vi "Version_2.0_Single_Column_Code.vi"() -> ()   [LabVIEW 2020] (continued)
                                n1436 = local read "VISA Refnum in\nfor Pump"() -> (w1853:refnum<visa-resource-name>)
                                n1437 = case shown="True" w1852 {
                                frame False {
                                }
                                frame True {
                                n1438 = local read "VISA Refnum in\nfor Pump"() -> (w1854:refnum<visa-resource-name>)
                                n1439 = call "HardStopCurrentProcess (SubVI).vi"("VISA Refnum in"=w1854) -> ()  [unwired: 11 in]
                                }
                                }
                                n1440 = call "ProcessCompletionWaiter (SubVI).vi"("VISA Refnum in"=w1853) -> ()  [unwired: 11 in]
                                }
                                }
                                }
                              }
                            }
                          }
                          frame #3 {
                            n1441 = local read "VISA Refnum in\nfor Pump"() -> (w1856:refnum<visa-resource-name>)
                            n1442 = local read "Port for \nB-Elution"() -> (w1855:string)
                            n1443 = call "PortChanger (SubVI).vi"("Port Number"=w1855, "VISA Refnum in"=w1856) -> ()  [unwired: 10 in]
                          }
                          frame #4 {
                            n1444 = local read "VISA Refnum in\nfor Pump"() -> (w1857:refnum<visa-resource-name>)
                            n1445 = call "ProcessCompletionWaiter (SubVI).vi"("VISA Refnum in"=w1857) -> ()  [unwired: 11 in]
                          }
                          frame #5 {
                            n1446 = local read "Buffer-B PickUp \nFlow Rate (ul/min)"() -> (w1860:dbl)
                            n1447 = local read "Buffer-B Pumping\nResolution"() -> (w1859:T2)
                            n1448 = local read "VISA Refnum in\nfor Pump"() -> (w1862:refnum<visa-resource-name>)
                            n1449 = local read "Buffer-B Volume \nto be  Pumped"() -> (w1858:dbl)
                            n1450 = local read "Volume of Syringe"() -> (w1861:dbl)
                            n1451 = call "RPickUp(SubVI).vi"("Volume to be picked up"=w1858, "Volume of Syringe"=w1861, "Resolution of PickUP"=w1859, "PickUp Flow Rate (ul/min)"=w1860, "VISA Refnum in"=w1862) -> ()  [unwired: 6 in, 1 out]
                          }
                          frame #6 {
                            n1452 = local read "Stopper that ends \nthe main loops"() -> (w1863:bool)
                            n1453 = local read "VISA Refnum in\nfor Pump"() -> (w1864:refnum<visa-resource-name>)
                            n1454 = case shown="True" w1863 {
                              frame False {
                              }
                              frame True {
                                n1455 = local read "VISA Refnum in\nfor Pump"() -> (w1865:refnum<visa-resource-name>)
                                n1456 = call "HardStopCurrentProcess (SubVI).vi"("VISA Refnum in"=w1865) -> ()  [unwired: 11 in]
                              }
                            }
                            n1457 = call "ProcessCompletionWaiter (SubVI).vi"("VISA Refnum in"=w1864) -> ()  [unwired: 11 in]
                          }
                          frame #7 {
                            # "Reads the initial Plunger Position for computing the volume dispensed"
                            n1458 = local read "VISA Refnum in\nfor Pump"() -> (w1867:refnum<visa-resource-name>)
                            n1459 = call "AbsolutePlungerPosition (SubVI).vi"("VISA Refnum in"=w1867) -> ("Plunger Position"=w1866:i32)  [unwired: 10 in]
                            n1460 = local write "Initial Plunger Position"(w1866) -> ()
                          }
                          frame #8 {
                            # "Switch to Port-2"
                            # "Port-2 of the pump is conncted to column-1 of chip"
                            n1461 = local read "VISA Refnum in\nfor Pump"() -> (w1869:refnum<visa-resource-name>)
                            n1462 = call "PortChanger (SubVI).vi"("Port Number"="2", "VISA Refnum in"=w1869) -> ()  [unwired: 10 in]
                          }
                          frame #9 {
                            n1463 = local read "Stopper that ends \nthe main loops"() -> (w1870:bool)
                            n1464 = local read "VISA Refnum in\nfor Pump"() -> (w1871:refnum<visa-resource-name>)
                            n1465 = case shown="True" w1870 {
                              frame False {
                              }
                              frame True {
                                n1466 = local read "VISA Refnum in\nfor Pump"() -> (w1872:refnum<visa-resource-name>)
                                n1467 = call "HardStopCurrentProcess (SubVI).vi"("VISA Refnum in"=w1872) -> ()  [unwired: 11 in]
                              }
                            }
                            n1468 = call "ProcessCompletionWaiter (SubVI).vi"("VISA Refnum in"=w1871) -> ()  [unwired: 11 in]
                          }
                          frame #10 {
                            # "Keeps the AMF valve after column-1 open and valve after column-2 closed"
                            n1469 = local read "VISA Refnum in\nfor Valve"() -> (w1877:refnum<visa-resource-name>)
                            n1470 = local read "External Valve \nOPEN"() -> (w1876:string)
                            n1471 = call "PortChanger_Valve (SubVI).vi"("Port Number"=w1876, "VISA Refnum in"=w1877) -> ()  [unwired: 10 in]
                            n1472 = local write "Valve V1 Open"(TRUE ("Valve V1 Open")) -> ()
                            n1473 = local write "Valve V2 Open"(TRUE ("Valve V2 Open")) -> ()
                            n1474 = local write "Valve V3 Open"(FALSE ("Valve V3 Open")) -> ()
                            n1475 = local write "Valve V4 Open"(FALSE ("Valve V4 Open")) -> ()
                            n1476 = local write "Valve V6 Open"(FALSE ("Valve V6 Open")) -> ()
                            n1477 = local write "Valve V5 Open"(FALSE ("Valve V5 Open")) -> ()
                            n1478 = local write "Valve V7 Open"(FALSE ("Valve V7 Open")) -> ()
                          }
                          frame #11 {
                            n1479 = local read "Buffer-B Dispense\nFlow Rate (ul/min)"() -> (w1887:dbl)
                            n1480 = local read "Buffer-B Pumping\nResolution"() -> (w1886:T2)
                            n1481 = local read "Initial Plunger Position"() -> (w1883:dbl)
                            n1482 = local read "VISA Refnum in\nfor Pump"() -> (w1889:refnum<visa-resource-name>)
                            n1483 = local read "Volume of Syringe"() -> (w1888:dbl)
                            n1484 = call "GoToAbsolutePosition(SubVI).vi"("Absolute Volume Position in Syringe (in ul)"=0.0 ("Volume to be Dispensed"), "Volume of Syringe"=w1888, "Resolution of Pumping"=w1886, "Flow Rate (ul/min)"=w1887, "VISA Refnum in"=w1889) -> ()  [unwired: 6 in, 1 out]
                            n1485 = local write "Pause Data Collection"(FALSE ("Pause Data Collection")) -> ()
                            n1486 = local write "Vol_now"(0.0 ("Vol_now")) -> ()
                            n1487 = local write "Position\nNow"(w1883) -> ()
                          }
                          frame #12 {
                            n1488 = while {
                              stop <- w1896 stop-if-true
                              n1489 = event shown="[1] Timeout" {
                                selector: _ -> [_ _]
                                dyn-events: _ -> [_ _]
                                timeout: 100 -> [_ _]
                                event "Pause Elution\nValue": Value Change {
                                n1490 = event-data() -> ()  [unwired: 1 in, 6 out]
                                n1491 = stacked-sequence {
                                frame #0 {
                                n1492 = local read "Pause Elution"() -> (w1898:bool)
                                n1493 = case shown="False" w1898 {
                                frame False {
                                n1494 = local write "Pause Elution"(TRUE ("Pause Elution")) -> ()
                                }
                                frame True {
                                n1495 = local write "Pause Elution"(FALSE ("Pause Elution")) -> ()
                                }
                                }
                                }
                                frame #1 {
                                n1496 = local read "Pause Elution"() -> (w1901:bool)
                                n1497 = case shown="False" w1901 {
                                frame False {
                                n1498 = local read "Buffer-B Dispense\nFlow Rate (ul/min)"() -> (w1906:dbl)
                                n1499 = local read "VISA Refnum in\nfor Pump"() -> (w1907:refnum<visa-resource-name>)
                                n1500 = local read "Buffer-B Pumping\nResolution"() -> (w1903:T2)
                                n1501 = local read "Volume of Syringe"() -> (w1904:dbl)
                                n1502 = call "GoToAbsolutePosition(SubVI).vi"("Absolute Volume Position in Syringe (in ul)"=0.0, "Volume of Syringe"=w1904, "Resolution of Pumping"=w1903, "Flow Rate (ul/min)"=w1906, "VISA Refnum in"=w1907) -> ()  [unwired: 6 in, 1 out]
                                n1503 = local write "Pause Data Collection"(FALSE ("Pause Data Collection")) -> ()
                                }
                                frame True {
                                n1504 = local read "VISA Refnum in\nfor Pump"() -> (w1909:refnum<visa-resource-name>)
                                n1505 = local write "Pause Data Collection"(TRUE ("Pause Data Collection")) -> ()
                                n1506 = call "HardStopCurrentProcess (SubVI).vi"("VISA Refnum in"=w1909) -> ()  [unwired: 11 in]
                                }
                                }
                                }
                                }
                                }
                                event Timeout {
                                n1507 = event-data() -> ()  [unwired: 1 in, 3 out]
                                }
                              }
                              n1508 = local read "Stopper that ends \nthe main loops"() -> (w1895:bool)
                              n1509 = local read "Divert Sample \ninto Column-2"() -> (w1894:bool)
                              n1510 = Or(x=w1894, y=w1895) -> (x .or. y?=w1896:bool)
                            }
                            n1511 = local read "Buffer-B Pumping\nResolution"() -> (w1892:T2)
                            n1512 = local read "VISA Refnum in\nfor Pump"() -> (w1893:refnum<visa-resource-name>)
                            n1513 = local read "Volume of Syringe"() -> (w1891:dbl)
                            n1514 = while {
                              tunnel: w1893 -> [w1918]
                              tunnel: w1892 -> [w1917]
                              tunnel: w1891 -> [w1916]
                              stop <- w1912 stop-if-true
                              n1515 = local read "Position\nNow"() -> (w1910:dbl)
                              n1516 = local read "Pause Elution"() -> (w1911:bool)
                              n1517 = case shown="True" w1911 {
                                tunnel: w1910 -> [w1922 _]
                                tunnel: w1918 -> [w1921 w1964]
                                tunnel: w1917 -> [w1920 _]
                                tunnel: w1916 -> [w1919 _]
                                frame False {
                                n1518 = stacked-sequence {
                                tunnel: w1922 -> [_ w1928]
                                tunnel: w1921 -> [_ w1927]
                                tunnel: w1920 -> [_ w1926]
                                tunnel: w1919 -> [_ w1925]
                                frame #0 {
                                n1519 = Wait (ms)(milliseconds to wait=u32 3000) -> ()  [unwired: 1 out]
                                n1520 = local write "Signal"(TRUE ("Signal")) -> ()
                                }
                                frame #1 {
                                n1521 = while {
                                tunnel: w1928 -> [w1940]
                                tunnel: w1927 -> [w1939]
                                tunnel: w1926 -> [w1938]
                                tunnel: w1925 -> [w1937]
                                stop <- w1932 stop-if-true
                                n1522 = stacked-sequence {
                                tunnel: w1940 -> [_ w1947]
                                tunnel: w1939 -> [_ w1946]
                                tunnel: w1938 -> [_ w1945]
                                tunnel: w1937 -> [_ w1944]
                                frame #0 {
                                n1523 = Wait (ms)(milliseconds to wait=u32 500) -> ()  [unwired: 1 out]
                                }
                                frame #1 {
                                n1524 = call "AbsolutePlungerPosition (SubVI).vi"("VISA Refnum in"=w1946) -> ("Plunger Position"=w1943:i32)  [unwired: 10 in]
                                n1525 = case shown="\"High Resolution Pumping\"" w1945 {
                                tunnel: w1947 -> [w1952 w1961]
                                tunnel: w1943 -> [w1953 w1960]
                                tunnel: [w1951 w1958] -> w1942
                                tunnel: w1944 -> [w1950 w1959]
                                frame "Standard Pumping", Default {
                                n1526 = Subtract(x=w1952, y=w1953) -> (x-y=w1949:dbl)
                                n1527 = Absolute Value(x=w1949) -> (abs(x)=w1948:dbl)
                                n1528 = Multiply(x=w1948, y=w1950) -> (x*y=w1955:dbl)
                                n1529 = Divide(x=w1955, y=3000.0) -> (x/y=w1951:dbl)
                                }
                                frame "High Resolution Pumping" {
                                n1530 = Subtract(x=w1961, y=w1960) -> (x-y=w1957:dbl)
                                n1531 = Absolute Value(x=w1957) -> (abs(x)=w1956:dbl)
                                n1532 = Multiply(x=w1956, y=w1959) -> (x*y=w1963:dbl)
                                n1533 = Divide(x=w1963, y=24000.0) -> (x/y=w1958:dbl)
                                }
                                }
                                n1534 = local write "Volume being Injected \nin this process"(w1942) -> ()
                                }
                                }
                                n1535 = local read "Volume being Injected \nin this process"() -> (w1930:dbl)
                                n1536 = local read "Affinity Elution \nGraph Min CutOff"() -> (w1929:dbl)
                                n1537 = local read "Stopper that ends \nthe main loops"() -> (w1935:bool)
                                n1538 = local read "Divert Sample \ninto Column-2"() -> (w1936:bool)
                                n1539 = Greater Or Equal?(x=w1930, y=w1929) -> (x >= y?=w1931:bool)
                                n1540 = Or(x=w1936, y=w1935) -> (x .or. y?=w1933:bool)
                                n1541 = local read "Pause Elution"() -> (w1934:bool)
                                n1542 = local write "Affinity Elution \nis Approaching"(w1931) -> ()
                                n1543 = Or(x=w1934, y=w1933) -> (x .or. y?=w1932:bool)
                                }
                                }
                                }
                                }
                                frame True {
                                n1544 = stacked-sequence {
                                tunnel: w1964 -> [_ w1967 _]
                                frame #0 {
                                n1545 = Wait (ms)(milliseconds to wait=u32 2000) -> ()  [unwired: 1 out]
                                }
                                frame #1 {
                                n1546 = local read "Signal"() -> (w1966:bool)
                                n1547 = case shown="True" w1966 {
                                tunnel: w1967 -> [_ w1973]
                                frame False {
                                }
                                frame True {
                                n1548 = local read "Volume being Injected \nin this process"() -> (w1971:dbl)
                                n1549 = local read "Net Elution \nVolume"() -> (w1970:dbl)
                                n1550 = local write "Signal"(FALSE ("Signal")) -> ()
                                n1551 = Add(x=w1971, y=w1970) -> (x+y=w1969:dbl)
                                n1552 = call "AbsolutePlungerPosition (SubVI).vi"("VISA Refnum in"=w1973) -> ("Plunger Position"=w1972:i32)  [unwired: 10 in]
                                n1553 = local write "Net Elution \nVolume"(w1969) -> ()
                                n1554 = local write "Position\nNow"(w1972) -> ()
                                }
                                }
                                }
                                frame #2 {
                                n1555 = local write "Volume being Injected \nin this process"(0.0 ("Volume being Injected \nin this process")) -> ()
                                }
                                }
                                }
                              }
                              n1556 = local read "Stopper that ends \nthe main loops"() -> (w1914:bool)
                              n1557 = local read "Divert Sample \ninto Column-2"() -> (w1913:bool)
                              n1558 = Or(x=w1913, y=w1914) -> (x .or. y?=w1912:bool)
                              n1559 = Wait (ms)(milliseconds to wait=u32 300) -> ()  [unwired: 1 out]
                            }
                            n1560 = local read "Stopper that ends \nthe main loops"() -> (w1890:bool)
                            n1561 = case shown="True" w1890 {
                              frame False {
                              }
                              frame True {
                                n1562 = local read "VISA Refnum in\nfor Pump"() -> (w1975:refnum<visa-resource-name>)
                                n1563 = call "HardStopCurrentProcess (SubVI).vi"("VISA Refnum in"=w1975) -> ()  [unwired: 11 in]
                              }
                            }
                          }
                          frame #13 {
                            # "valve after column-1 is closed"
                            # "Keeps the on-chip Valve V1 and V3 after column-2 open"
                            # "Keeps the AMF valve after column-1 closed and valve after column-2 open"
                            n1564 = local read "VISA Refnum in\nfor Pump"() -> (w1988:refnum<visa-resource-name>)
                            n1565 = local read "Volume being Injected \nin this process"() -> (w1985:dbl)
                            n1566 = local write "Sample Volume Diverted\ninto Column-2"(0.0 ("Sample Volume Diverted\ninto Column-2")) -> ()
                            n1567 = call "AbsolutePlungerPosition (SubVI).vi"("VISA Refnum in"=w1988) -> ("Plunger Position"=w1987:i32)  [unwired: 10 in]
                            n1568 = local write "Position\nNow"(w1987) -> ()
                            n1569 = local write "Vol_previous"(0.0 ("Vol_diff")) -> ()
                            n1570 = local write "Vol_now"(w1985) -> ()
                            n1571 = local read "VISA Refnum in\nfor Valve"() -> (w1980:refnum<visa-resource-name>)
                            n1572 = local read "External Valve \nCLOSED"() -> (w1979:string)
                            n1573 = local write "Valve V1 Open"(TRUE ("Valve V1 Open")) -> ()
                            n1574 = local write "Valve V3 Open"(TRUE ("Valve V3 Open")) -> ()
                            n1575 = local write "Valve V2 Open"(FALSE ("Valve V2 Open")) -> ()
                            n1576 = local write "Valve V4 Open"(TRUE ("Valve V4 Open")) -> ()
                            n1577 = call "PortChanger_Valve (SubVI).vi"("Port Number"=w1979, "VISA Refnum in"=w1980) -> ()  [unwired: 10 in]
                            n1578 = local write "Valve V5 Open"(TRUE ("Valve V5 Open")) -> ()
                            n1579 = local write "Valve V6 Open"(FALSE ("Valve V6 Open")) -> ()
                            n1580 = local write "Valve V7 Open"(TRUE ("Valve V7 Open")) -> ()
                          }
                          frame #14 {
                            n1581 = local read "Divert Sample \ninto Column-2"() -> (w1990:bool)
                            n1582 = case shown="True" w1990 {
                              frame False {
                                n1583 = stacked-sequence {
                                frame #0 {
                                n1584 = local read "Buffer-B Pumping\nResolution"() -> (w1993:T2)
                                n1585 = local read "VISA Refnum in\nfor Pump"() -> (w1995:refnum<visa-resource-name>)
                                n1586 = local read "Initial Plunger Position"() -> (w1994:dbl)
                                n1587 = local read "Volume of Syringe"() -> (w1992:dbl)
                                n1588 = while {
                                tunnel: w1994 -> [w2001]
                                tunnel: w1995 -> [w2000]
                                tunnel: w1993 -> [w1999]
                                tunnel: w1992 -> [w1998]
                                stop <- w1996 stop-if-true
                                n1589 = Wait (ms)(milliseconds to wait=u32 100) -> ()  [unwired: 1 out]
                                n1590 = stacked-sequence {
                                tunnel: w2001 -> [w2007 _]
                                tunnel: w2000 -> [w2006 w2027]
                                tunnel: w1999 -> [w2005 _]
                                tunnel: w1998 -> [w2004 _]
                                tunnel: [_ w2025] -> w1996
                                frame #0 {
                                n1591 = call "AbsolutePlungerPosition (SubVI).vi"("VISA Refnum in"=w2006) -> ("Plunger Position"=w2003:i32)  [unwired: 10 in]
                                n1592 = case shown="\"Standard Pumping\", Default" w2005 {
                                tunnel: w2007 -> [w2012 w2021]
                                tunnel: w2003 -> [w2013 w2020]
                                tunnel: [w2011 w2018] -> w2002
                                tunnel: w2004 -> [w2010 w2019]
                                frame "Standard Pumping", Default {
                                n1593 = Subtract(x=w2012, y=w2013) -> (x-y=w2009:dbl)
                                n1594 = Absolute Value(x=w2009) -> (abs(x)=w2008:dbl)
                                n1595 = Multiply(x=w2008, y=w2010) -> (x*y=w2015:dbl)
                                n1596 = Divide(x=w2015, y=3000.0) -> (x/y=w2011:dbl)
                                }
                                frame "High Resolution Pumping" {
                                n1597 = Subtract(x=w2021, y=w2020) -> (x-y=w2017:dbl)
                                n1598 = Absolute Value(x=w2017) -> (abs(x)=w2016:dbl)
                                n1599 = Multiply(x=w2016, y=w2019) -> (x*y=w2023:dbl)
                                n1600 = Divide(x=w2023, y=24000.0) -> (x/y=w2018:dbl)
                                }
                                }
                                n1601 = local write "Volume being Injected \nin this process"(w2002) -> ()
                                }
                                frame #1 {
                                n1602 = local read "Stopper that ends \nthe main loops"() -> (w2024:bool)
                                n1603 = call "LSPOneStatus (SubVI).vi"("VISA Refnum in"=w2027) -> ("read buffer"=w2029:string)  [unwired: 10 in]
                                n1604 = call <vilib>:"Trim Whitespace.vi"("string"=w2029) -> ("trimmed string"=w2028:string)  [unwired: 1 in]
                                n1605 = Equal?(x=w2028, y="/0`\u0003") -> (x = y?=w2026:bool)
                                n1606 = Or(x=w2026, y=w2024) -> (x .or. y?=w2025:bool)
                                }
                                }
                                }
                                n1607 = local read "Stopper that ends \nthe main loops"() -> (w1991:bool)
                                n1608 = case shown="True" w1991 {
                                frame False {
                                }
                                frame True {
                                n1609 = local read "VISA Refnum in\nfor Pump"() -> (w2031:refnum<visa-resource-name>)
                                n1610 = call "HardStopCurrentProcess (SubVI).vi"("VISA Refnum in"=w2031) -> ()  [unwired: 11 in]
                                }
                                }
                                }
                                }
                              }
                              frame True {
                                n1611 = stacked-sequence {
                                frame #0 {
                                n1612 = local read "Buffer-B Pumping\nResolution"() -> (w2034:T2)
                                n1613 = local read "VISA Refnum in\nfor Pump"() -> (w2036:refnum<visa-resource-name>)
                                n1614 = local read "Volume of Syringe"() -> (w2033:dbl)
                                n1615 = local read "Position\nNow"() -> (w2035:dbl)
                                n1616 = while {
                                tunnel: w2035 -> [w2042]
                                tunnel: w2036 -> [w2041]
                                tunnel: w2034 -> [w2040]
                                tunnel: w2033 -> [w2039]
                                stop <- w2037 stop-if-true
                                n1617 = Wait (ms)(milliseconds to wait=u32 100) -> ()  [unwired: 1 out]
                                n1618 = stacked-sequence {
                                tunnel: w2042 -> [w2052 _ _]
                                tunnel: w2041 -> [w2051 _ w2078]
                                tunnel: w2040 -> [w2050 _ _]
                                tunnel: w2039 -> [w2049 _ _]
                                tunnel: [_ _ w2076] -> w2037
                                frame #0 {
                                n1619 = local read "Vol_previous"() -> (w2046:dbl)
                                n1620 = call "AbsolutePlungerPosition (SubVI).vi"("VISA Refnum in"=w2051) -> ("Plunger Position"=w2048:i32)  [unwired: 10 in]
                                n1621 = case shown="\"Standard Pumping\", Default" w2050 {
                                tunnel: w2052 -> [w2057 w2066]
                                tunnel: w2048 -> [w2058 w2065]
                                tunnel: [w2056 w2063] -> w2047
                                tunnel: w2049 -> [w2055 w2064]
                                frame "Standard Pumping", Default {
                                n1622 = Subtract(x=w2057, y=w2058) -> (x-y=w2054:dbl)
                                n1623 = Absolute Value(x=w2054) -> (abs(x)=w2053:dbl)
                                n1624 = Multiply(x=w2053, y=w2055) -> (x*y=w2060:dbl)
                                n1625 = Divide(x=w2060, y=3000.0) -> (x/y=w2056:dbl)
                                }
                                frame "High Resolution Pumping" {
                                n1626 = Subtract(x=w2066, y=w2065) -> (x-y=w2062:dbl)
                                n1627 = Absolute Value(x=w2062) -> (abs(x)=w2061:dbl)
                                n1628 = Multiply(x=w2061, y=w2064) -> (x*y=w2068:dbl)
                                n1629 = Divide(x=w2068, y=24000.0) -> (x/y=w2063:dbl)
                                }
                                }
                                n1630 = Subtract(x=w2047, y=w2046) -> (x-y=w2045:dbl)
                                n1631 = local read "Vol_now"() -> (w2043:dbl)
                                n1632 = local write "Sample Volume Diverted\ninto Column-2"(w2047) -> ()
                                n1633 = Add(x=w2045, y=w2043) -> (x+y=w2044:dbl)
                                n1634 = local write "Volume being Injected \nin this process"(w2044) -> ()
                                }
                                frame #1 {
                                n1635 = local read "Volume being Injected \nin this process"() -> (w2069:dbl)
                                n1636 = local read "Sample Volume Diverted\ninto Column-2"() -> (w2070:dbl)
                                n1637 = local write "Vol_now"(w2069) -> ()
                                n1638 = local write "Vol_previous"(w2070) -> ()
                                }
                                frame #2 {
                                n1639 = local read "Buffer-B Volume \nto be Pumped for\nSample Diversion\nto Column-2"() -> (w2072:dbl)
                                n1640 = local read "Sample Volume Diverted\ninto Column-2"() -> (w2071:dbl)
                                n1641 = local read "Stopper that ends \nthe main loops"() -> (w2073:bool)
                                n1642 = call "LSPOneStatus (SubVI).vi"("VISA Refnum in"=w2078) -> ("read buffer"=w2080:string)  [unwired: 10 in]
                                n1643 = call <vilib>:"Trim Whitespace.vi"("string"=w2080) -> ("trimmed string"=w2079:string)  [unwired: 1 in]
                                n1644 = Equal?(x=w2079, y="/0`\u0003") -> (x = y?=w2077:bool)
                                n1645 = Greater Or Equal?(x=w2071, y=w2072) -> (x >= y?=w2075:bool)
                                n1646 = Or(x=w2073, y=w2075) -> (x .or. y?=w2074:bool)
                                n1647 = Or(x=w2077, y=w2074) -> (x .or. y?=w2076:bool)
                                }
                                }
                                }
                                n1648 = local read "Stopper that ends \nthe main loops"() -> (w2032:bool)
                                n1649 = case shown="True" w2032 {
                                frame False {
                                }
                                frame True {
                                n1650 = local read "VISA Refnum in\nfor Pump"() -> (w2082:refnum<visa-resource-name>)
                                n1651 = call "HardStopCurrentProcess (SubVI).vi"("VISA Refnum in"=w2082) -> ()  [unwired: 11 in]
                                }
                                }
                                }
                                frame #1 {
                                n1652 = local read "VISA Refnum in\nfor Pump"() -> (w2084:refnum<visa-resource-name>)
                                n1653 = local write "Pause Data Collection"(TRUE ("Pause Data Collection")) -> ()
                                n1654 = call "HardStopCurrentProcess (SubVI).vi"("VISA Refnum in"=w2084) -> ()  [unwired: 11 in]
                                }
                                frame #2 {
                                n1655 = local read "VISA Refnum in\nfor Pump"() -> (w2085:refnum<visa-resource-name>)
                                n1656 = call "PortChanger (SubVI).vi"("Port Number"="1", "VISA Refnum in"=w2085) -> ()  [unwired: 10 in]
                                }
                                frame #3 {
                                n1657 = local read "VISA Refnum in\nfor Pump"() -> (w2091:refnum<visa-resource-name>)
                                n1658 = local read "Volume of Syringe"() -> (w2087:dbl)
                                n1659 = call "GoToAbsolutePosition(SubVI).vi"("Absolute Volume Position in Syringe (in ul)"=0.0, "Volume of Syringe"=w2087, "Resolution of Pumping"=T2."Standard Pumping", "Flow Rate (ul/min)"=150.0, "VISA Refnum in"=w2091) -> ()  [unwired: 6 in, 1 out]
                                }
                                frame #4 {
                                n1660 = local read "VISA Refnum in\nfor Pump"() -> (w2093:refnum<visa-resource-name>)
                                n1661 = local write "Divert Sample \ninto Column-2"(FALSE ("Divert Sample \ninto Column-2")) -> ()
                                n1662 = call "ProcessCompletionWaiter (SubVI).vi"("VISA Refnum in"=w2093) -> ()  [unwired: 11 in]
                                }
                                }
                              }
                            }
                          }
                          frame #15 {
                            # "Keeps the On-Chip Valves V1 and V3 closed"
                            # "Switch to Port-5/8"
                            # "Port-5/8 of pump is connected to Buffer-C1/C2"
                            # "Keeps the AMF valve after column-1 open and valve after column-2 closed"
                            n1663 = local read "VISA Refnum in\nfor Pump"() -> (w2106:refnum<visa-resource-name>)
                            n1664 = local write "Pause Data Collection"(TRUE ("Pause Data Collection")) -> ()
                            n1665 = Wait (ms)(milliseconds to wait=u32 500) -> ()  [unwired: 1 out]
                            n1666 = local write "Affinity On"(FALSE ("Affinity On")) -> ()
                            n1667 = local read "Port for \nC2-Elution"() -> (w2097:string)
                            n1668 = local write "Affinity Elution On"(FALSE ("Affinity Elution On")) -> ()
                            n1669 = call "PortChanger (SubVI).vi"("Port Number"=w2097, "VISA Refnum in"=w2106) -> ()  [unwired: 10 in]
                            n1670 = local read "VISA Refnum in\nfor Valve"() -> (w2100:refnum<visa-resource-name>)
                            n1671 = local read "External Valve \nCLOSED"() -> (w2099:string)
                            n1672 = local write "Valve V1 Open"(FALSE ("Valve V1 Open")) -> ()
                            n1673 = local write "Valve V2 Open"(FALSE ("Valve V2 Open")) -> ()
                            n1674 = local write "Valve V3 Open"(FALSE ("Valve V3 Open")) -> ()
                            n1675 = local write "Valve V4 Open"(FALSE ("Valve V4 Open")) -> ()
                            n1676 = call "PortChanger_Valve (SubVI).vi"("Port Number"=w2099, "VISA Refnum in"=w2100) -> ()  [unwired: 10 in]
                            n1677 = local write "Valve V5 Open"(FALSE ("Valve V5 Open")) -> ()
                            n1678 = local write "Valve V6 Open"(FALSE ("Valve V6 Open")) -> ()
                            n1679 = local write "Valve V7 Open"(FALSE ("Valve V7 Open")) -> ()
                          }
                          frame #16 {
                            n1680 = local read "VISA Refnum in\nfor Pump"() -> (w2110:refnum<visa-resource-name>)
                            n1681 = call "ProcessCompletionWaiter (SubVI).vi"("VISA Refnum in"=w2110) -> ()  [unwired: 11 in]
                            n1682 = local write "Start the Process"(FALSE ("Start the Process")) -> ()
                          }
                          frame #17 {
                            n1683 = local read "Stopper that ends \nthe main loops"() -> (w2114:bool)
                            n1684 = local read "Start the Process"() -> (w2115:bool)
                            n1685 = Or(x=w2115, y=w2114) -> (x .or. y?=w2113:bool)
                            n1686 = local write "Elution of Column-1"(FALSE ("Elution of Column-1")) -> ()
                            n1687 = case shown="False" w2113 {
                              frame False {
                                n1688 = while {
                                stop <- w2119 stop-if-true
                                n1689 = local read "Stopper that ends \nthe main loops"() -> (w2120:bool)
                                n1690 = local read "Start the Process"() -> (w2121:bool)
                                n1691 = Or(x=w2121, y=w2120) -> (x .or. y?=w2119:bool)
                                n1692 = Wait (ms)(milliseconds to wait=u32 10) -> ()  [unwired: 1 out]
                                }
                                n1693 = One Button Dialog(message="Move to Column-2 detection zone and Press 'Start the Process' Button.") -> ()  [unwired: 1 in, 1 out]
                              }
                              frame True {
                              }
                            }
                            n1694 = local write "Volume being Injected \nin this process"(0.0 ("Volume being Injected \nin this process")) -> ()
                            n1695 = local write "Elution of Column-2"(TRUE ("Elution of Column-2")) -> ()
                          }
                          frame #18 {
                            # "If Yes, it will clean the SEC buffer from port-8 tubing else it will clean the pump valve a bit"
                            n1696 = local read "Clean the \nBuffer-C2 tubing"() -> (w2122:bool)
                            n1697 = case shown="False" w2122 {
                              frame False {
                                n1698 = stacked-sequence {
                                frame #0 {
                                n1699 = local read "VISA Refnum in\nfor Pump"() -> (w2124:refnum<visa-resource-name>)
                                n1700 = local read "Port for \nC2-Elution"() -> (w2123:string)
                                n1701 = call "PortChanger (SubVI).vi"("Port Number"=w2123, "VISA Refnum in"=w2124) -> ()  [unwired: 10 in]
                                }
                                frame #1 {
                                n1702 = local read "VISA Refnum in\nfor Pump"() -> (w2125:refnum<visa-resource-name>)
                                n1703 = call "ProcessCompletionWaiter (SubVI).vi"("VISA Refnum in"=w2125) -> ()  [unwired: 11 in]
                                }
                                frame #2 {
                                n1704 = local read "Buffer-C2 Pumping\nResolution"() -> (w2128:T2)
                                n1705 = local read "VISA Refnum in\nfor Pump"() -> (w2130:refnum<visa-resource-name>)
                                n1706 = local read "V-S"() -> (w2126:dbl)
                                n1707 = local read "Volume of Syringe"() -> (w2129:dbl)
                                n1708 = call "RPickUp(SubVI).vi"("Volume to be picked up"=w2126, "Volume of Syringe"=w2129, "Resolution of PickUP"=w2128, "PickUp Flow Rate (ul/min)"=150.0, "VISA Refnum in"=w2130) -> ()  [unwired: 6 in, 1 out]
                                }
                                frame #3 {
                                n1709 = local read "Stopper that ends \nthe main loops"() -> (w2131:bool)
                                n1710 = local read "VISA Refnum in\nfor Pump"() -> (w2132:refnum<visa-resource-name>)
                                n1711 = case shown="True" w2131 {
                                frame False {
                                }
                                frame True {
                                n1712 = local read "VISA Refnum in\nfor Pump"() -> (w2133:refnum<visa-resource-name>)
                                n1713 = call "HardStopCurrentProcess (SubVI).vi"("VISA Refnum in"=w2133) -> ()  [unwired: 11 in]
                                }
                                }
                                n1714 = call "ProcessCompletionWaiter (SubVI).vi"("VISA Refnum in"=w2132) -> ()  [unwired: 11 in]
                                }
                                frame #4 {
                                n1715 = local read "VISA Refnum in\nfor Pump"() -> (w2135:refnum<visa-resource-name>)
                                n1716 = call "PortChanger (SubVI).vi"("Port Number"="1", "VISA Refnum in"=w2135) -> ()  [unwired: 10 in]
                                }
                                frame #5 {
                                n1717 = local read "Stopper that ends \nthe main loops"() -> (w2136:bool)
                                n1718 = local read "VISA Refnum in\nfor Pump"() -> (w2137:refnum<visa-resource-name>)
                                n1719 = case shown="True" w2136 {
                                frame False {
                                }
                                frame True {
                                n1720 = local read "VISA Refnum in\nfor Pump"() -> (w2138:refnum<visa-resource-name>)
                                n1721 = call "HardStopCurrentProcess (SubVI).vi"("VISA Refnum in"=w2138) -> ()  [unwired: 11 in]
                                }
                                }
                                n1722 = call "ProcessCompletionWaiter (SubVI).vi"("VISA Refnum in"=w2137) -> ()  [unwired: 11 in]
                                }
                                frame #6 {
                                n1723 = local read "VISA Refnum in\nfor Pump"() -> (w2143:refnum<visa-resource-name>)
                                n1724 = local read "Volume of Syringe"() -> (w2140:dbl)
                                n1725 = call "GoToAbsolutePosition(SubVI).vi"("Absolute Volume Position in Syringe (in ul)"=0.0, "Volume of Syringe"=w2140, "Resolution of Pumping"=T2."Standard Pumping", "Flow Rate (ul/min)"=150.0, "VISA Refnum in"=w2143) -> ()  [unwired: 6 in, 1 out]
                                }
                                frame #7 {
                                n1726 = local read "Stopper that ends \nthe main loops"() -> (w2144:bool)
                                n1727 = local read "VISA Refnum in\nfor Pump"() -> (w2145:refnum<visa-resource-name>)
                                n1728 = case shown="True" w2144 {
                                frame False {
                                }
                                frame True {
                                n1729 = local read "VISA Refnum in\nfor Pump"() -> (w2146:refnum<visa-resource-name>)
                                n1730 = call "HardStopCurrentProcess (SubVI).vi"("VISA Refnum in"=w2146) -> ()  [unwired: 11 in]
                                }
                                }
                                n1731 = call "ProcessCompletionWaiter (SubVI).vi"("VISA Refnum in"=w2145) -> ()  [unwired: 11 in]
                                }
                                }
                              }
                              frame True {
                                n1732 = for {
                                N: 2 -> [_]
                                n1733 = stacked-sequence {
                                frame #0 {
                                n1734 = local read "VISA Refnum in\nfor Pump"() -> (w2149:refnum<visa-resource-name>)
                                n1735 = local read "Port for \nC2-Elution"() -> (w2148:string)
                                n1736 = call "PortChanger (SubVI).vi"("Port Number"=w2148, "VISA Refnum in"=w2149) -> ()  [unwired: 10 in]
                                }
                                frame #1 {
                                n1737 = local read "VISA Refnum in\nfor Pump"() -> (w2150:refnum<visa-resource-name>)
                                n1738 = call "ProcessCompletionWaiter (SubVI).vi"("VISA Refnum in"=w2150) -> ()  [unwired: 11 in]
                                }
                                frame #2 {
                                n1739 = local read "Buffer-C2 Pumping\nResolution"() -> (w2153:T2)
                                n1740 = local read "VISA Refnum in\nfor Pump"() -> (w2155:refnum<visa-resource-name>)
                                n1741 = local read "Apparent Volume\nof Syringe"() -> (w2151:dbl)
                                n1742 = local read "Volume of Syringe"() -> (w2154:dbl)
                                n1743 = call "RPickUp(SubVI).vi"("Volume to be picked up"=w2151, "Volume of Syringe"=w2154, "Resolution of PickUP"=w2153, "PickUp Flow Rate (ul/min)"=150.0, "VISA Refnum in"=w2155) -> ()  [unwired: 6 in, 1 out]
                                }
                                frame #3 {
                                n1744 = local read "Stopper that ends \nthe main loops"() -> (w2156:bool)
                                n1745 = local read "VISA Refnum in\nfor Pump"() -> (w2157:refnum<visa-resource-name>)
                                n1746 = case shown="True" w2156 {
                                frame False {
                                }
                                frame True {
                                n1747 = local read "VISA Refnum in\nfor Pump"() -> (w2158:refnum<visa-resource-name>)
                                n1748 = call "HardStopCurrentProcess (SubVI).vi"("VISA Refnum in"=w2158) -> ()  [unwired: 11 in]
                                }
                                }
                                n1749 = call "ProcessCompletionWaiter (SubVI).vi"("VISA Refnum in"=w2157) -> ()  [unwired: 11 in]
                                }
                                frame #4 {
                                n1750 = local read "VISA Refnum in\nfor Pump"() -> (w2160:refnum<visa-resource-name>)
                                n1751 = call "PortChanger (SubVI).vi"("Port Number"="1", "VISA Refnum in"=w2160) -> ()  [unwired: 10 in]
                                }
                                frame #5 {
                                n1752 = local read "Stopper that ends \nthe main loops"() -> (w2161:bool)
                                n1753 = local read "VISA Refnum in\nfor Pump"() -> (w2162:refnum<visa-resource-name>)
                                n1754 = case shown="True" w2161 {
                                frame False {
                                }
                                frame True {
                                n1755 = local read "VISA Refnum in\nfor Pump"() -> (w2163:refnum<visa-resource-name>)
                                n1756 = call "HardStopCurrentProcess (SubVI).vi"("VISA Refnum in"=w2163) -> ()  [unwired: 11 in]
                                }
                                }
                                n1757 = call "ProcessCompletionWaiter (SubVI).vi"("VISA Refnum in"=w2162) -> ()  [unwired: 11 in]
                                }
                                frame #6 {
                                n1758 = local read "VISA Refnum in\nfor Pump"() -> (w2168:refnum<visa-resource-name>)
                                n1759 = local read "Volume of Syringe"() -> (w2165:dbl)
                                n1760 = call "GoToAbsolutePosition(SubVI).vi"("Absolute Volume Position in Syringe (in ul)"=0.0, "Volume of Syringe"=w2165, "Resolution of Pumping"=T2."Standard Pumping", "Flow Rate (ul/min)"=150.0, "VISA Refnum in"=w2168) -> ()  [unwired: 6 in, 1 out]
                                }
                                frame #7 {
                                n1761 = local read "Stopper that ends \nthe main loops"() -> (w2169:bool)
                                n1762 = local read "VISA Refnum in\nfor Pump"() -> (w2170:refnum<visa-resource-name>)
                                n1763 = case shown="True" w2169 {
                                frame False {
                                }
                                frame True {
                                n1764 = local read "VISA Refnum in\nfor Pump"() -> (w2171:refnum<visa-resource-name>)
                                n1765 = call "HardStopCurrentProcess (SubVI).vi"("VISA Refnum in"=w2171) -> ()  [unwired: 11 in]
                                }
                                }
                                n1766 = call "ProcessCompletionWaiter (SubVI).vi"("VISA Refnum in"=w2170) -> ()  [unwired: 11 in]
                                }
                                }
                                }
                              }
                            }
                          }
                          frame #19 {
                            n1767 = local read "VISA Refnum in\nfor Pump"() -> (w2173:refnum<visa-resource-name>)
                            n1768 = local read "Port for \nC2-Elution"() -> (w2172:string)
                            n1769 = call "PortChanger (SubVI).vi"("Port Number"=w2172, "VISA Refnum in"=w2173) -> ()  [unwired: 10 in]
                          }
                          frame #20 {
                            n1770 = local read "VISA Refnum in\nfor Pump"() -> (w2174:refnum<visa-resource-name>)
                            n1771 = call "ProcessCompletionWaiter (SubVI).vi"("VISA Refnum in"=w2174) -> ()  [unwired: 11 in]
                          }
                          frame #21 {
                            n1772 = local read "Buffer-C2 PickUp \nFlow Rate (ul/min)"() -> (w2178:dbl)
                            n1773 = local read "Buffer-C2 Pumping\nResolution"() -> (w2177:T2)
                            n1774 = local read "VISA Refnum in\nfor Pump"() -> (w2180:refnum<visa-resource-name>)
                            n1775 = local read "Buffer-C2 Volume \nto be Pumped"() -> (w2176:dbl)
                            n1776 = local read "Volume of Syringe"() -> (w2179:dbl)
                            n1777 = call "RPickUp(SubVI).vi"("Volume to be picked up"=w2176, "Volume of Syringe"=w2179, "Resolution of PickUP"=w2177, "PickUp Flow Rate (ul/min)"=w2178, "VISA Refnum in"=w2180) -> ()  [unwired: 6 in, 1 out]
                            n1778 = local write "SEC On"(TRUE ("SEC On")) -> ()
                          }
                          frame #22 {
                            n1779 = local read "Stopper that ends \nthe main loops"() -> (w2181:bool)
                            n1780 = local read "VISA Refnum in\nfor Pump"() -> (w2182:refnum<visa-resource-name>)
                            n1781 = case shown="True" w2181 {
                              frame False {
                              }
                              frame True {
                                n1782 = local read "VISA Refnum in\nfor Pump"() -> (w2183:refnum<visa-resource-name>)
                                n1783 = call "HardStopCurrentProcess (SubVI).vi"("VISA Refnum in"=w2183) -> ()  [unwired: 11 in]
                              }
                            }
                            n1784 = call "ProcessCompletionWaiter (SubVI).vi"("VISA Refnum in"=w2182) -> ()  [unwired: 11 in]
                          }
                          frame #23 {
                            # "Reads the initial Plunger Position for computing the volume dispensed"
                            n1785 = local read "VISA Refnum in\nfor Pump"() -> (w2185:refnum<visa-resource-name>)
                            n1786 = call "AbsolutePlungerPosition (SubVI).vi"("VISA Refnum in"=w2185) -> ("Plunger Position"=w2184:i32)  [unwired: 10 in]
                            n1787 = local write "Initial Plunger Position"(w2184) -> ()
                          }
                          frame #24 {
                            # "Switch to Port-10"
                            # "Port-10 of the pump is conncted to column-2 of chip"
                            n1788 = local read "VISA Refnum in\nfor Pump"() -> (w2187:refnum<visa-resource-name>)
                            n1789 = call "PortChanger (SubVI).vi"("Port Number"="10", "VISA Refnum in"=w2187) -> ()  [unwired: 10 in]
                          }
                          frame #25 {
                            n1790 = local read "Stopper that ends \nthe main loops"() -> (w2188:bool)
                            n1791 = local read "VISA Refnum in\nfor Pump"() -> (w2189:refnum<visa-resource-name>)
                            n1792 = case shown="True" w2188 {
                              frame False {
                              }
                              frame True {
                                n1793 = local read "VISA Refnum in\nfor Pump"() -> (w2190:refnum<visa-resource-name>)
                                n1794 = call "HardStopCurrentProcess (SubVI).vi"("VISA Refnum in"=w2190) -> ()  [unwired: 11 in]
                              }
                            }
                            n1795 = call "ProcessCompletionWaiter (SubVI).vi"("VISA Refnum in"=w2189) -> ()  [unwired: 11 in]
                          }
                          frame #26 {
                            # "Keeps the AMF valve after column-1 open and valve after column-2 closed"
                            n1796 = local read "Buffer-C2 Dispense\nFlow Rate (ul/min)"() -> (w2203:dbl)
                            n1797 = local read "Buffer-C2 Pumping\nResolution"() -> (w2202:T2)
                            n1798 = local read "VISA Refnum in\nfor Pump"() -> (w2205:refnum<visa-resource-name>)
                            n1799 = local write "Pause Data Collection"(FALSE ("Pause Data Collection")) -> ()
                            n1800 = local read "Volume of Syringe"() -> (w2204:dbl)
                            n1801 = call "GoToAbsolutePosition(SubVI).vi"("Absolute Volume Position in Syringe (in ul)"=0.0 ("Volume to be Dispensed"), "Volume of Syringe"=w2204, "Resolution of Pumping"=w2202, "Flow Rate (ul/min)"=w2203, "VISA Refnum in"=w2205) -> ()  [unwired: 6 in, 1 out]
                            n1802 = local read "VISA Refnum in\nfor Valve"() -> (w2199:refnum<visa-resource-name>)
                            n1803 = local read "External Valve \nOPEN"() -> (w2198:string)
                            n1804 = local write "Valve V1 Open"(FALSE ("Valve V1 Open")) -> ()
                            n1805 = local write "Valve V2 Open"(TRUE ("Valve V2 Open")) -> ()
                            n1806 = local write "Valve V3 Open"(TRUE ("Valve V3 Open")) -> ()
                            n1807 = local write "Valve V4 Open"(FALSE ("Valve V4 Open")) -> ()
                            n1808 = call "PortChanger_Valve (SubVI).vi"("Port Number"=w2198, "VISA Refnum in"=w2199) -> ()  [unwired: 10 in]
                            n1809 = local write "Valve V5 Open"(FALSE ("Valve V5 Open")) -> ()
                            n1810 = local write "Valve V6 Open"(FALSE ("Valve V6 Open")) -> ()
                            n1811 = local write "Valve V7 Open"(FALSE ("Valve V7 Open")) -> ()
                          }
                          frame #27 {
                            n1812 = local read "Initial Plunger Position"() -> (w2209:dbl)
                            n1813 = local read "Buffer-C2 Pumping\nResolution"() -> (w2208:T2)
                            n1814 = local read "VISA Refnum in\nfor Pump"() -> (w2210:refnum<visa-resource-name>)
                            n1815 = local read "Volume of Syringe"() -> (w2207:dbl)
                            n1816 = while {
                              tunnel: w2209 -> [w2216]
                              tunnel: w2210 -> [w2215]
                              tunnel: w2208 -> [w2214]
                              tunnel: w2207 -> [w2213]
                              stop <- w2211 stop-if-true
                              n1817 = Wait (ms)(milliseconds to wait=u32 100) -> ()  [unwired: 1 out]
                              n1818 = stacked-sequence {
                                tunnel: w2216 -> [w2222 _]
                                tunnel: w2215 -> [w2221 w2248]
                                tunnel: w2214 -> [w2220 _]
                                tunnel: w2213 -> [w2219 _]
                                tunnel: [_ w2244] -> w2211
                                frame #0 {
                                n1819 = call "AbsolutePlungerPosition (SubVI).vi"("VISA Refnum in"=w2221) -> ("Plunger Position"=w2218:i32)  [unwired: 10 in]
                                n1820 = case shown="\"Standard Pumping\", Default" w2220 {
                                tunnel: w2222 -> [w2227 w2236]
                                tunnel: w2218 -> [w2228 w2235]
                                tunnel: [w2226 w2233] -> w2217
                                tunnel: w2219 -> [w2225 w2234]
                                frame "Standard Pumping", Default {
                                n1821 = Subtract(x=w2227, y=w2228) -> (x-y=w2224:dbl)
                                n1822 = Absolute Value(x=w2224) -> (abs(x)=w2223:dbl)
                                n1823 = Multiply(x=w2223, y=w2225) -> (x*y=w2230:dbl)
                                n1824 = Divide(x=w2230, y=3000.0) -> (x/y=w2226:dbl)
                                }
                                frame "High Resolution Pumping" {
                                n1825 = Subtract(x=w2236, y=w2235) -> (x-y=w2232:dbl)
                                n1826 = Absolute Value(x=w2232) -> (abs(x)=w2231:dbl)
                                n1827 = Multiply(x=w2231, y=w2234) -> (x*y=w2238:dbl)
                                n1828 = Divide(x=w2238, y=24000.0) -> (x/y=w2233:dbl)
                                }
                                }
                                n1829 = local write "Volume being Injected \nin this process"(w2217) -> ()
                                }
                                frame #1 {
                                n1830 = local read "Stopper that ends \nthe main loops"() -> (w2245:bool)
                                n1831 = local read "Divert Buffer-C \ninto Column-2"() -> (w2246:bool)
                                n1832 = local read "Volume being Injected \nin this process"() -> (w2243:dbl)
                                n1833 = call "LSPOneStatus (SubVI).vi"("VISA Refnum in"=w2248) -> ("read buffer"=w2250:string)  [unwired: 10 in]
                                n1834 = call <vilib>:"Trim Whitespace.vi"("string"=w2250) -> ("trimmed string"=w2249:string)  [unwired: 1 in]
                                n1835 = Equal?(x=w2249, y="/0`\u0003") -> (x = y?=w2247:bool)
                                n1836 = Or(x=w2246, y=w2245) -> (x .or. y?=w2241:bool)
                                n1837 = Greater Or Equal?(x=w2243, y=2.0) -> (x >= y?=w2240:bool)
                                n1838 = Or(x=w2241, y=w2240) -> (x .or. y?=w2239:bool)
                                n1839 = Or(x=w2247, y=w2239) -> (x .or. y?=w2244:bool)
                                }
                              }
                            }
                            n1840 = local read "Stopper that ends \nthe main loops"() -> (w2206:bool)
                            n1841 = case shown="True" w2206 {
                              frame False {
                              }
                              frame True {
                                n1842 = local read "VISA Refnum in\nfor Pump"() -> (w2252:refnum<visa-resource-name>)
                                n1843 = call "HardStopCurrentProcess (SubVI).vi"("VISA Refnum in"=w2252) -> ()  [unwired: 11 in]
                              }
                            }
                          }
                          frame #28 {
                            # "Keeps the on-chip valves V4, V5 and V7 open"
                            # "Keeps the AMF valve after column-1 closed and valve after column-2 open"
                            n1844 = local write "Divert Buffer-C \ninto Column-2"(FALSE ("Divert Buffer-C \ninto Column-2")) -> ()
                            n1845 = local read "VISA Refnum in\nfor Pump"() -> (w2257:refnum<visa-resource-name>)
                            n1846 = local read "External Valve \nCLOSED"() -> (w2256:string)
                            n1847 = local write "Valve V3 Open"(FALSE ("Valve V3 Open")) -> ()
                            n1848 = local write "Valve V2 Open"(FALSE ("Valve V2 Open")) -> ()
                            n1849 = local write "Valve V1 Open"(FALSE ("Valve V1 Open")) -> ()
                            n1850 = local write "Valve V4 Open"(TRUE ("Valve V4 Open")) -> ()
                            n1851 = call "PortChanger_Valve (SubVI).vi"("Port Number"=w2256, "VISA Refnum in"=w2257) -> ()  [unwired: 10 in]
                            n1852 = local write "Valve V5 Open"(TRUE ("Valve V5 Open")) -> ()
                            n1853 = local write "Valve V6 Open"(FALSE ("Valve V6 Open")) -> ()
                            n1854 = local write "Valve V7 Open"(TRUE ("Valve V7 Open")) -> ()
                          }
                          frame #29 {
                            n1855 = local read "Initial Plunger Position"() -> (w2266:dbl)
                            n1856 = local read "Buffer-C2 Pumping\nResolution"() -> (w2265:T2)
                            n1857 = local read "VISA Refnum in\nfor Pump"() -> (w2267:refnum<visa-resource-name>)
                            n1858 = local read "Volume of Syringe"() -> (w2264:dbl)
                            n1859 = while {
                              tunnel: w2266 -> [w2273]
                              tunnel: w2267 -> [w2272]
                              tunnel: w2265 -> [w2271]
                              tunnel: w2264 -> [w2270]
                              stop <- w2268 stop-if-true
                              n1860 = Wait (ms)(milliseconds to wait=u32 100) -> ()  [unwired: 1 out]
                              n1861 = stacked-sequence {
                                tunnel: w2273 -> [w2279 _]
                                tunnel: w2272 -> [w2278 w2301]
                                tunnel: w2271 -> [w2277 _]
                                tunnel: w2270 -> [w2276 _]
                                tunnel: [_ w2299] -> w2268
                                frame #0 {
                                n1862 = call "AbsolutePlungerPosition (SubVI).vi"("VISA Refnum in"=w2278) -> ("Plunger Position"=w2275:i32)  [unwired: 10 in]
                                n1863 = case shown="\"Standard Pumping\", Default" w2277 {
                                tunnel: w2279 -> [w2284 w2293]
                                tunnel: w2275 -> [w2285 w2292]
                                tunnel: [w2283 w2290] -> w2274
                                tunnel: w2276 -> [w2282 w2291]
                                frame "Standard Pumping", Default {
                                n1864 = Subtract(x=w2284, y=w2285) -> (x-y=w2281:dbl)
                                n1865 = Absolute Value(x=w2281) -> (abs(x)=w2280:dbl)
                                n1866 = Multiply(x=w2280, y=w2282) -> (x*y=w2287:dbl)
                                n1867 = Divide(x=w2287, y=3000.0) -> (x/y=w2283:dbl)
                                }
                                frame "High Resolution Pumping" {
                                n1868 = Subtract(x=w2293, y=w2292) -> (x-y=w2289:dbl)
                                n1869 = Absolute Value(x=w2289) -> (abs(x)=w2288:dbl)
                                n1870 = Multiply(x=w2288, y=w2291) -> (x*y=w2295:dbl)
                                n1871 = Divide(x=w2295, y=24000.0) -> (x/y=w2290:dbl)
                                }
                                }
                                n1872 = local write "Volume being Injected \nin this process"(w2274) -> ()
                                }
                                frame #1 {
                                n1873 = call "LSPOneStatus (SubVI).vi"("VISA Refnum in"=w2301) -> ("read buffer"=w2303:string)  [unwired: 10 in]
                                n1874 = call <vilib>:"Trim Whitespace.vi"("string"=w2303) -> ("trimmed string"=w2302:string)  [unwired: 1 in]
                                n1875 = Equal?(x=w2302, y="/0`\u0003") -> (x = y?=w2300:bool)
                                n1876 = local read "Stopper that ends \nthe main loops"() -> (w2297:bool)
                                n1877 = local read "Divert Sample \nonto Grid"() -> (w2298:bool)
                                n1878 = Or(x=w2298, y=w2297) -> (x .or. y?=w2296:bool)
                                n1879 = Or(x=w2300, y=w2296) -> (x .or. y?=w2299:bool)
                                }
                              }
                            }
                            n1880 = local read "Stopper that ends \nthe main loops"() -> (w2263:bool)
                            n1881 = case shown="True" w2263 {
                              frame False {
                              }
                              frame True {
                                n1882 = local read "VISA Refnum in\nfor Pump"() -> (w2305:refnum<visa-resource-name>)
                                n1883 = call "HardStopCurrentProcess (SubVI).vi"("VISA Refnum in"=w2305) -> ()  [unwired: 11 in]
                              }
                            }
                          }
                          frame #30 {
                            n1884 = local read "Volume being Injected \nin this process"() -> (w2308:dbl)
                            n1885 = local read "VISA Refnum in\nfor Pump"() -> (w2310:refnum<visa-resource-name>)
                            n1886 = call "AbsolutePlungerPosition (SubVI).vi"("VISA Refnum in"=w2310) -> ("Plunger Position"=w2309:i32)  [unwired: 10 in]
                            n1887 = local write "Pause Data Collection"(TRUE) -> ()
                            n1888 = local write "True Volume being \ninjected in this\nprocess"(w2308) -> ()
                            n1889 = local write "Position\nNow"(w2309) -> ()
                            n1890 = Wait (ms)(milliseconds to wait=u32 500) -> ()  [unwired: 1 out]
                          }
                          frame #31 {
                            # "Sample Deposition onto EM-Grid"
                            n1891 = local read "Divert Sample \nonto Grid"() -> (w2311:bool)
                            n1892 = case shown="True" w2311 {
                              frame False {
                              }
                              frame True {
                                n1893 = stacked-sequence {
                                frame #0 {
                                # "Discard the initial volume of fluid that is present in the channel prior to detection"
                                n1894 = local read "Buffer-C2 Pumping\nResolution"() -> (w2322:T2)
                                n1895 = local read "Initial Plunger Position"() -> (w2321:dbl)
                                n1896 = local read "VISA Refnum in\nfor Pump"() -> (w2323:refnum<visa-resource-name>)
                                n1897 = local read "Position\nNow"() -> (w2319:dbl)
                                n1898 = local read "Volume of Syringe"() -> (w2320:dbl)
                                n1899 = local write "Pause Data Collection"(FALSE) -> ()
                                n1900 = while {
                                tunnel: w2323 -> [w2333]
                                tunnel: w2322 -> [w2332]
                                tunnel: w2321 -> [w2328]
                                tunnel: w2320 -> [w2331]
                                tunnel: w2319 -> [w2327]
                                stop <- w2329 stop-if-true
                                n1901 = stacked-sequence {
                                tunnel: w2333 -> [w2339 w2361 w2391]
                                tunnel: w2332 -> [w2338 w2360 _]
                                tunnel: w2328 -> [w2336 _ _]
                                tunnel: w2331 -> [w2335 w2358 _]
                                tunnel: [_ _ w2384] -> w2329
                                tunnel: w2327 -> [_ w2356 _]
                                frame #0 {
                                # "From here on 'True Volume being injected \nin this process' represents the true total \nvolume in this process"
                                n1902 = call "AbsolutePlungerPosition (SubVI).vi"("VISA Refnum in"=w2339) -> ("Plunger Position"=w2337:i32)  [unwired: 10 in]
                                n1903 = case shown="..\"Standard Pumping\"" w2338 {
                                tunnel: w2337 -> [w2347 w2355]
                                tunnel: w2336 -> [w2346 w2354]
                                tunnel: w2335 -> [w2343 w2351]
                                tunnel: [w2340 w2348] -> w2334
                                frame .."Standard Pumping" {
                                n1904 = Subtract(x=w2347, y=w2346) -> (x-y=w2345:dbl)
                                n1905 = Absolute Value(x=w2345) -> (abs(x)=w2344:dbl)
                                n1906 = Multiply(x=w2344, y=w2343) -> (x*y=w2342:dbl)
                                n1907 = Divide(x=w2342, y=3000.0) -> (x/y=w2340:dbl)
                                }
                                frame "High Resolution Pumping".. {
                                n1908 = Subtract(x=w2355, y=w2354) -> (x-y=w2353:dbl)
                                n1909 = Absolute Value(x=w2353) -> (abs(x)=w2352:dbl)
                                n1910 = Multiply(x=w2352, y=w2351) -> (x*y=w2350:dbl)
                                n1911 = Divide(x=w2350, y=24000.0) -> (x/y=w2348:dbl)
                                }
                                }
                                n1912 = local write "True Volume being \ninjected in this\nprocess"(w2334) -> ()
                                }
                                frame #1 {
                                # "From here on 'Volume being injected \nin this process' represents the volume \nin this sub process"
                                n1913 = call "AbsolutePlungerPosition (SubVI).vi"("VISA Refnum in"=w2361) -> ("Plunger Position"=w2359:i32)  [unwired: 10 in]
                                n1914 = case shown="..\"Standard Pumping\"" w2360 {
                                tunnel: w2359 -> [w2369 w2377]
                                tunnel: w2356 -> [w2368 w2376]
                                tunnel: w2358 -> [w2365 w2373]
                                tunnel: [w2362 w2370] -> w2357
                                frame .."Standard Pumping" {
                                n1915 = Subtract(x=w2369, y=w2368) -> (x-y=w2367:dbl)
                                n1916 = Absolute Value(x=w2367) -> (abs(x)=w2366:dbl)
                                n1917 = Multiply(x=w2366, y=w2365) -> (x*y=w2364:dbl)
                                n1918 = Divide(x=w2364, y=3000.0) -> (x/y=w2362:dbl)
                                }
                                frame "High Resolution Pumping".. {
                                n1919 = Subtract(x=w2377, y=w2376) -> (x-y=w2375:dbl)
                                n1920 = Absolute Value(x=w2375) -> (abs(x)=w2374:dbl)
                                n1921 = Multiply(x=w2374, y=w2373) -> (x*y=w2372:dbl)
                                n1922 = Divide(x=w2372, y=24000.0) -> (x/y=w2370:dbl)
                                }
                                }
                                n1923 = local write "Volume being Injected \nin this process"(w2357) -> ()
                                }
                                frame #2 {
                                n1924 = local read "Discard Volume"() -> (w2378:dbl)
                                n1925 = local read "Discard fluid \nprior to 1st \ndeposition"() -> (w2383:bool)
                                n1926 = local read "Volume being Injected \nin this process"() -> (w2382:dbl)
                                n1927 = Greater Or Equal?(x=w2382, y=w2378) -> (x >= y?=w2380:bool)
                                n1928 = call "AbsolutePlungerPositionStatus (SubVI).vi"("VISA Refnum in"=w2391) -> ("read buffer"=w2390:string)  [unwired: 10 in]
                                n1929 = local read "Stop for End of \nExperiment \nand Data Writing"() -> (w2387:bool)
                                n1930 = call <vilib>:"Trim Whitespace.vi"("string"=w2390) -> ("trimmed string"=w2389:string)  [unwired: 1 in]
                                n1931 = Not(x=w2383) -> (.not. x?=w2381:bool)
                                n1932 = Equal?(x=w2389, y="/0`\u0003") -> (x = y?=w2386:bool)
                                n1933 = Or(x=w2381, y=w2380) -> (x .or. y?=w2379:bool)
                                n1934 = Or(x=w2379, y=w2387) -> (x .or. y?=w2385:bool)
                                n1935 = Or(x=w2386, y=w2385) -> (x .or. y?=w2384:bool)
                                }
                                }
                                n1936 = Wait (ms)(milliseconds to wait=u32 100) -> ()  [unwired: 1 out]
                                }
                                n1937 = local write "Valve V4 Open"(TRUE ("Valve V4 Open")) -> ()
                                n1938 = local write "Valve V3 Open"(FALSE ("Valve V3 Open")) -> ()
                                n1939 = local write "Valve V2 Open"(FALSE ("Valve V2 Open")) -> ()
                                n1940 = local write "Valve V1 Open"(FALSE ("Valve V1 Open")) -> ()
                                n1941 = local write "Valve V5 Open"(TRUE ("Valve V5 Open")) -> ()
                                n1942 = local write "Valve V6 Open"(TRUE ("Valve V6 Open")) -> ()
                                n1943 = local write "Valve V7 Open"(FALSE ("Valve V7 Open")) -> ()
                                n1944 = local write "Volume being Injected \nin this process"(0.0) -> ()
                                }
                                frame #1 {
                                # "Keeps the on-chip valve V1, V2 and V3 closed,\nHalts also deposition onto the grid\nand waits for the 1st redeposit command. Once the command is issued\nit starts pumpoing and moves onto the next frame"
                                n1945 = stacked-sequence {
                                frame #0 {
                                n1946 = local write "Valve V5 Open"(FALSE ("Valve V5 Open")) -> ()
                                n1947 = local write "Valve V1 Open"(FALSE ("Valve V1 Open")) -> ()
                                n1948 = local read "VISA Refnum in\nfor Pump"() -> (w2401:refnum<visa-resource-name>)
                                n1949 = local write "Valve V2 Open"(FALSE ("Valve V2 Open")) -> ()
                                n1950 = local write "Valve V6 Open"(FALSE ("Valve V6 Open")) -> ()
                                n1951 = local write "Re-deposit Sample\nonto Grid"(FALSE ("Redeposit Sample\nonto Grid")) -> ()
                                n1952 = local write "Pause Data Collection"(TRUE ("Pause Data Collection")) -> ()
                                n1953 = call "HardStopCurrentProcess (SubVI).vi"("VISA Refnum in"=w2401) -> ()  [unwired: 11 in]
                                n1954 = local write "Valve V7 Open"(FALSE ("Valve V7 Open")) -> ()
                                n1955 = local write "Valve V3 Open"(FALSE ("Valve V3 Open")) -> ()
                                n1956 = local write "Valve V4 Open"(FALSE ("Valve V4 Open")) -> ()
                                }
                                frame #1 {
                                n1957 = while {
                                stop <- w2404 stop-if-true
                                n1958 = local read "Stop for End of \nExperiment \nand Data Writing"() -> (w2405:bool)
                                n1959 = local read "Re-deposit Sample\nonto Grid"() -> (w2406:bool)
                                n1960 = Or(x=w2406, y=w2405) -> (x .or. y?=w2404:bool)
                                }
                                n1961 = local write "Discard fluid \nprior to 1st \ndeposition"(FALSE ("Discard fluid \nprior to 1st \ndeposition")) -> ()
                                n1962 = One Button Dialog(message="Do you want to deposit sample on another grid? If yes, turn on 'Re-deposit Sample onto Grid'. Else turn on STOP ") -> ()  [unwired: 1 in, 1 out]
                                }
                                frame #2 {
                                n1963 = local write "Valve V6 Open"(TRUE ("Valve V3 Open")) -> ()
                                n1964 = local write "Valve V4 Open"(TRUE ("Valve V1 Open")) -> ()
                                n1965 = local write "Valve V5 Open"(TRUE ("Valve V2 Open")) -> ()
                                n1966 = local write "Valve V7 Open"(FALSE ("Valve V7 Open")) -> ()
                                }
                                frame #3 {
                                n1967 = local read "Re-deposit Sample\nonto Grid"() -> (w2411:bool)
                                n1968 = case shown="True" w2411 {
                                frame False {
                                n1969 = local write "Suction On/Off"(FALSE ("Suction On/Off")) -> ()
                                }
                                frame True {
                                n1970 = stacked-sequence {
                                frame #0 {
                                n1971 = local read "VISA Refnum in\nfor Pump"() -> (w2414:refnum<visa-resource-name>)
                                n1972 = call "AbsolutePlungerPosition (SubVI).vi"("VISA Refnum in"=w2414) -> ("Plunger Position"=w2413:i32)  [unwired: 10 in]
                                n1973 = local write "Position\nNow"(w2413) -> ()
                                }
                                frame #1 {
                                n1974 = local read "Buffer-C2 Pumping\nResolution"() -> (w2416:T2)
                                n1975 = case shown="\"Standard Pumping\", Default" w2416 {
                                tunnel: [w2417 w2428] -> w2415
                                frame "Standard Pumping", Default {
                                n1976 = local read "Buffer-C2 Volume \nto be Pumped"() -> (w2420:dbl)
                                n1977 = local read "Volume of Syringe"() -> (w2423:dbl)
                                n1978 = local read "Initial Plunger Position"() -> (w2427:dbl)
                                n1979 = local read "Position\nNow"() -> (w2426:dbl)
                                n1980 = Subtract(x=w2427, y=w2426) -> (x-y=w2425:dbl)
                                n1981 = Absolute Value(x=w2425) -> (abs(x)=w2424:dbl)
                                n1982 = Multiply(x=w2424, y=w2423) -> (x*y=w2422:dbl)
                                n1983 = Divide(x=w2422, y=3000.0) -> (x/y=w2419:dbl)
